vi "Init.vi"(8 "error in (no error)":errorcluster, 11 "reference in":refnum<class "Login_Dialog.lvclass">) -> (0 "error out":errorcluster, 3 "reference out":refnum<class "Login_Dialog.lvclass">)   [LabVIEW 2022 SP3, in "Login_Dialog.lvlib" / "Login_Dialog.lvclass"]
uses:
  Login_Dialog.lvclass
  <vilib>/Utility/file.llb/Read Delimited Spreadsheet (string).vi
  Components/Login_Base.lvlibp/Login_Base.lvclass
  Components/ViPER.lvlibp/ViPER.lvclass
  C:/Projects/Medulla/ViPER/Examples/Flux_Capacitor_Tester/Components/ViPER.lvlibp/ViPER.lvclass
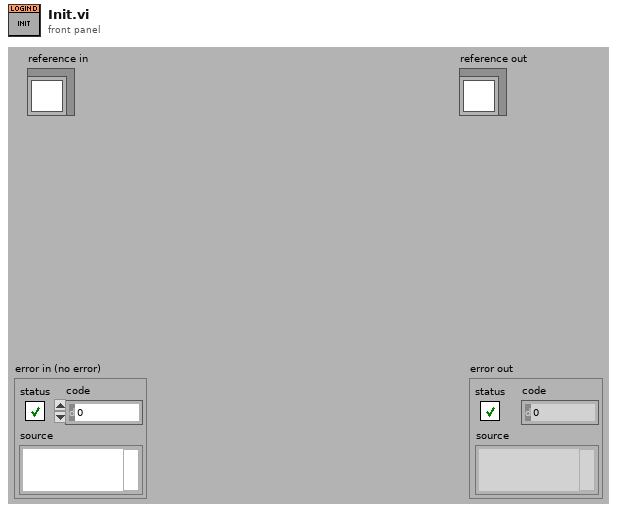
[diagram p1: front panel]
types:
  T1 = typedef "Login_Dialog.lvlib/Login_Dialog.lvclass/ObjectAttributes.ctl" = cluster{"Config":T2, "User":string, "LoggedIn":bool, "Users":string[][]}
  T2 = typedef "Login_Dialog.lvlib/Login_Dialog.lvclass/Config.ctl" = cluster{"default":string}
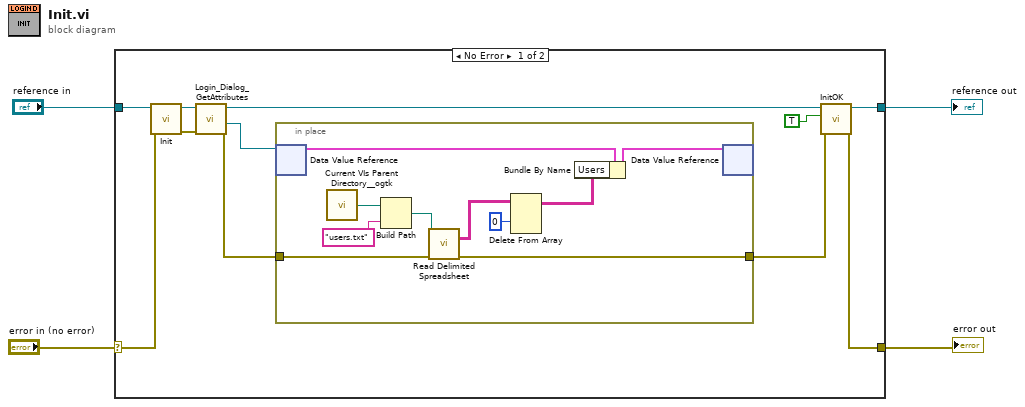
[diagram p0: block diagram]
diagram:
  n1 = case shown="No Error" "error in (no error)" {
    selector: "error in (no error)" -> [w14 w27]
    tunnel: [w5 w27] -> w3
    tunnel: [w8 w26] -> w1
    tunnel: "reference in" -> [w15 w26]
    frame No Error {
      n2 = call-parent "Init.vi"("error in (no error)"=w14, "reference in"=w15) -> ("error out"=w12:errorcluster, "reference out"=w13:refnum<class "Login_Dialog.lvclass">)  [unwired: 8 in]
      n3 = call "Login_Dialog_GetAttributes.vi"("error in (no error)"=w12, "reference in"=w13) -> ("error out"=w10:errorcluster, "DataRef"=w11:refnum<data-value>, "reference out"=w9:refnum<class "Login_Dialog.lvclass">)  [unwired: 6 in, 1 out]
      n4 = in-place {
        in-place-border: w10 -> [w25]
        in-place-border: [w24] -> w6
        n5 = in-place-dvr #1(w11) -> (w18:T1)  [unwired: 1 out]
        n6 = call <userlib>:"Current VIs Parent Directory__ogtk.vi"() -> ("Parent Directory (+ Relative)"=w23:path)  [unwired: 5 in]
        n7 = Build Path(base path=w23, name or relative path="users.txt") -> (appended path=w21:path)
        n8 = call-poly <vilib>:"Read Delimited Spreadsheet.vi"("file path (dialog if empty)"=w21, "error in (no error)"=w25) -> ("all rows"=w20:string[][], "error out"=w24:errorcluster)  [unwired: 8 in, 4 out]
        n9 = Delete From Array(array=w20, index (row)=0) -> (array with subset deleted=w16:string[][])  [unwired: 2 in, 1 out]
        n10 = Bundle By Name(cluster=w18, "Users"=w16) -> (w17:T1)
        n11 = in-place-dvr #1(w17) -> ()  [unwired: 2 out]
      }
      n12 = call "InitOK.vi"("error in (no error)"=w6, "Init OK?"=TRUE, "reference in"=w9) -> ("error out"=w5:errorcluster, "reference out"=w8:refnum<class "Login_Dialog.lvclass">)  [unwired: 7 in]
    }
    frame Error {
    }
  }
  "error out" <- w3
  "reference out" <- w1
